vi "Init.vi"(7 "Clust Refnum":refnum<vi>, 8 "error in (no error)":errorcluster, 9 "All_info":string[][](array[string]), 10 "Path_out":string[](array[string]), 11 "Data":T1) -> (0 "error out":errorcluster, 3 "Data Out":T1)   [LabVIEW 2014]
uses:
  controls/Data1.ctl
  controls/Payjson.ctl
panel:
  in  "Save Path":string="C:\\CS-BarCode\\Save Date\\"
  in  "IO Path":path=path "C:/CS-BarCode/Setting Data/Com.ini"
  in  "Model Path":path=path "C:/CS-BarCode/Setting Data/Model.csv"
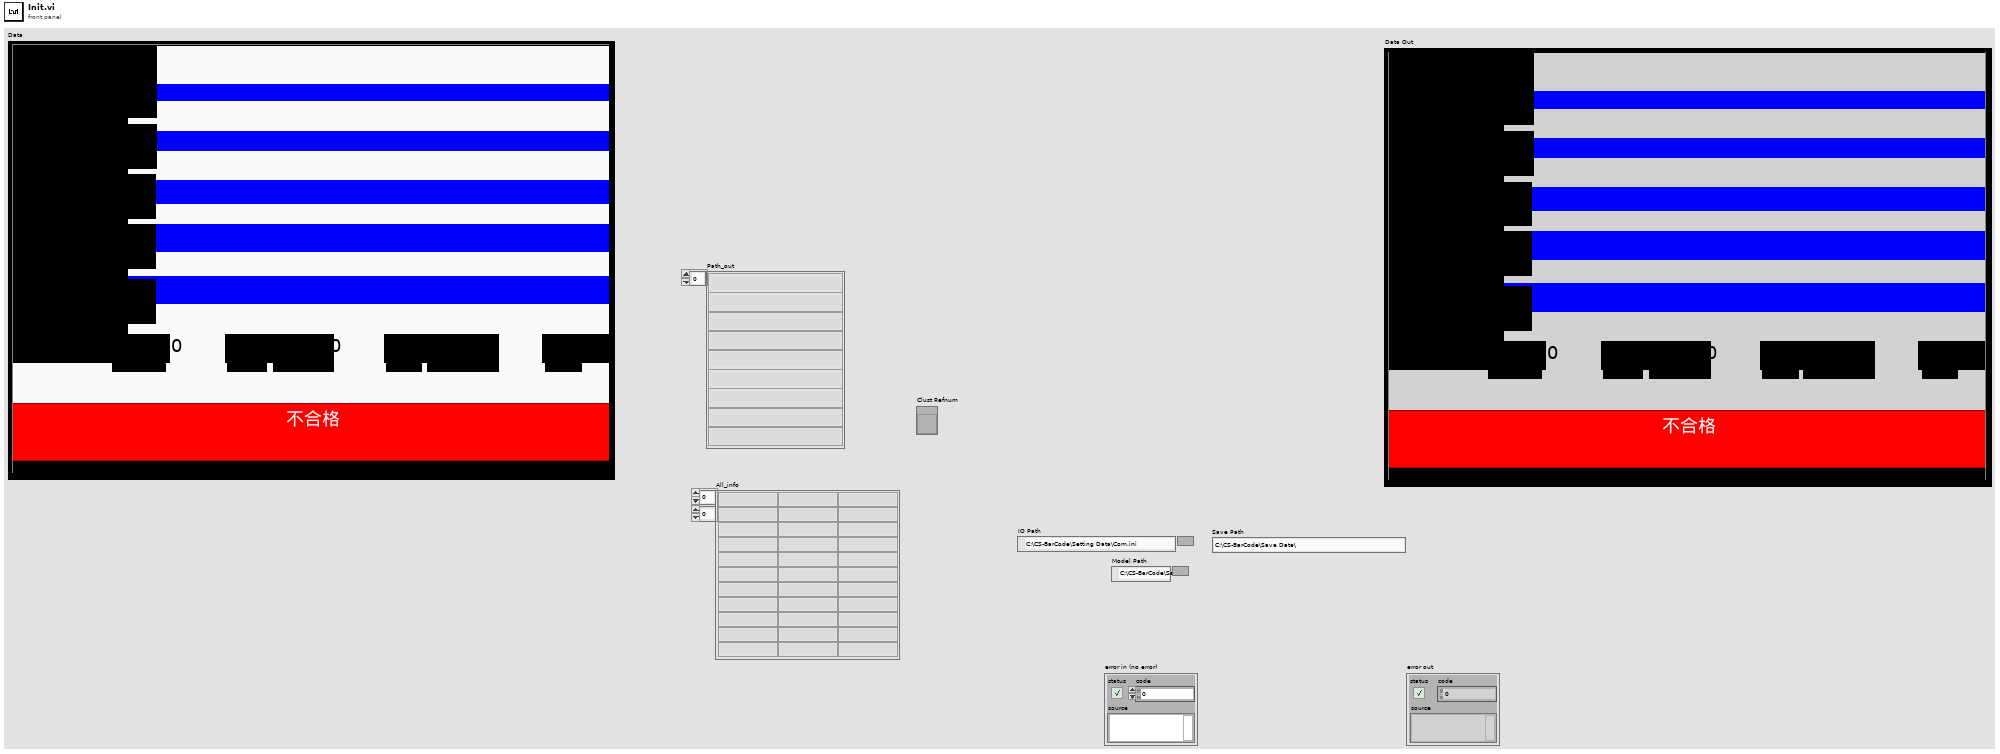
[diagram p1: front panel]
types:
  T1 = typedef "Data1.ctl" = cluster{"Date":string, "BarCode1":string, "BarCode2":string, "BarCode3":string, "Message":string, "OK Count":u16, "NG Count":u16, "Total Count":u16, "ModelData":string[][], "OK&NG":bool, "COM1":refnum<visa-resource-name>, "COM2":refnum<visa-resource-name>, "IO":i32, "Time":u32, "TCP":refnum<k5>, "TCP 2":refnum<k5>, "COM1 2":refnum<visa-resource-name>, "CheckNum":string, "BarCode1_1":string, "BarCode2_1":string, "BarCode3_1":string, "日期":string, "機種":string, "機號":string, "商品條碼1":string, "OK_1":string, "OK":string, "NG":string, "NG_1":string, "Total":string, "Total_1":string, "ClaerTime":u32, "Pjson":T2, "LotNo":string[], "CheckParsArray":string[], "BarCode4":string, "BarCode4_1":string, "商品條碼2":string, "BarCode5":string, "BarCode5_1":string, "商品條碼3":string, "ReScanNG":i32, "NGTimeCT":u32}
  T2 = typedef "Payjson.ctl" = cluster{"DEPT":string, "LINE":string, "STANO":string, "WORKNO":string, "PRODSN":string, "COMPNTID":string, "COMPNTLOT":string, "COMPNTSN":string, "USEDQTY":i16, "OPDATE":string, "OPUSER":string, "RECVDATE":string, "MMODU":string}[]
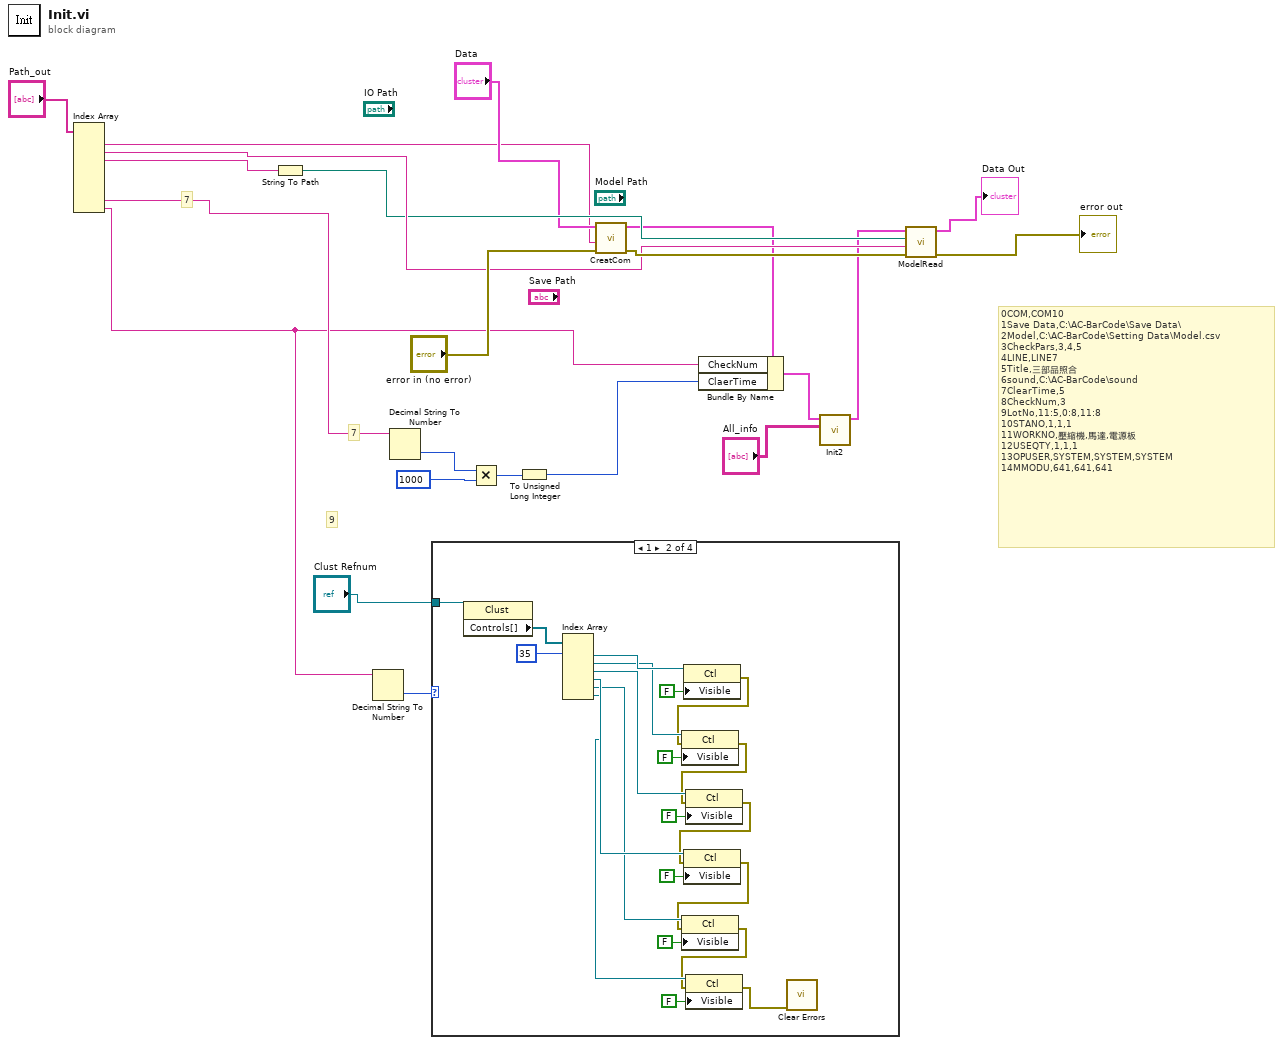
[diagram p0: block diagram]
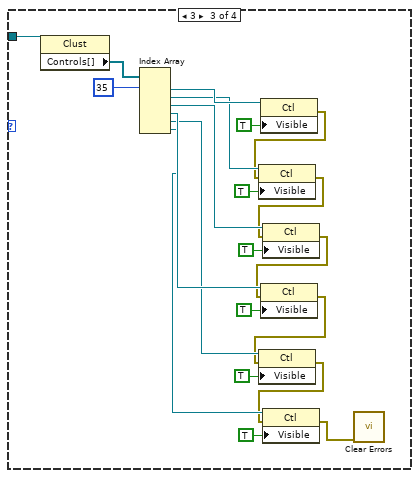
[diagram p3: hidden frame]
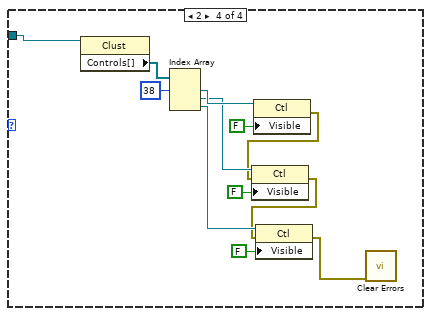
[diagram p4: hidden frame]
diagram:
  # "0COM,COM10\n1Save Data,C:\\AC-BarCode\\Save Data\\\n2Model,C:\\AC-BarCode\\Setting Data\\Model.csv\n3CheckPars,3,4,5\n4LINE,LINE7\n5Title,三部品照合\n6sound,C:\\AC-BarCode\\sound\n7ClearTime,5\n8CheckNum,3\n9LotNo,11:5,0:8,11:8\n10STANO,1,1,1\n11WORKNO,壓縮機,馬達,電源板\n12USEQTY,1,1,1\n13OPUSER,SYSTEM,SYSTEM,SYSTEM\n14MMODU,641,641,641"
  # "9"
  # "7"
  # "7"
  n1 = Index Array(array="Path_out") -> (element #1=w14:string, element #2=w18:string, element #3=w17:string, element #8=w13:string, element #9=w1:string)  [unwired: 9 in, 4 out]
  n2 = String To Path(string=w17) -> (path=w16:path)
  n3 = Decimal String To Number(string=w1) -> (number=w3:i32)  [unwired: 2 in, 1 out]
  n4 = Decimal String To Number(string=w13) -> (number=w12:i32)  [unwired: 2 in, 1 out]
  n5 = case shown="1" w3 {
    tunnel: "Clust Refnum" -> [_ w35 w56 w72]
    frame 0, Default {
    }
    frame 1 {
      n6 = property class="Clust"(reference=w35) -> ("Controls[]"=w43:refnum<vi>[])  [unwired: 1 in, 2 out]
      n7 = Index Array(array=w43, index #1=35 ("index")) -> (element #1=w41:refnum<vi>, element #2=w37:refnum<vi>, element #3=w36:refnum<vi>, element #4=w31:refnum<vi>, element #5=w30:refnum<vi>, element #6=w29:refnum<vi>)  [unwired: 5 in]
      n8 = property class="Ctl"(reference=w41, "Visible"=FALSE) -> (error out=w28:errorcluster)  [unwired: 1 in, 1 out]
      n9 = property class="Ctl"(reference=w37, error in=w28, "Visible"=FALSE) -> (error out=w27:errorcluster)  [unwired: 1 out]
      n10 = property class="Ctl"(reference=w36, error in=w27, "Visible"=FALSE) -> (error out=w26:errorcluster)  [unwired: 1 out]
      n11 = property class="Ctl"(reference=w31, error in=w26, "Visible"=FALSE) -> (error out=w25:errorcluster)  [unwired: 1 out]
      n12 = property class="Ctl"(reference=w30, error in=w25, "Visible"=FALSE) -> (error out=w24:errorcluster)  [unwired: 1 out]
      n13 = property class="Ctl"(reference=w29, error in=w24, "Visible"=FALSE) -> (error out=w23:errorcluster)  [unwired: 1 out]
      n14 = call <vilib>:"Clear Errors.vi"("error in (no error)"=w23) -> ()  [unwired: 5 in, 2 out]
    }
    frame 3 {
      n15 = property class="Clust"(reference=w56) -> ("Controls[]"=w64:refnum<vi>[])  [unwired: 1 in, 2 out]
      n16 = Index Array(array=w64, index #1=35 ("index")) -> (element #1=w62:refnum<vi>, element #2=w58:refnum<vi>, element #3=w57:refnum<vi>, element #4=w52:refnum<vi>, element #5=w51:refnum<vi>, element #6=w50:refnum<vi>)  [unwired: 5 in]
      n17 = property class="Ctl"(reference=w62, "Visible"=TRUE) -> (error out=w49:errorcluster)  [unwired: 1 in, 1 out]
      n18 = property class="Ctl"(reference=w58, error in=w49, "Visible"=TRUE) -> (error out=w48:errorcluster)  [unwired: 1 out]
      n19 = property class="Ctl"(reference=w57, error in=w48, "Visible"=TRUE) -> (error out=w47:errorcluster)  [unwired: 1 out]
      n20 = property class="Ctl"(reference=w52, error in=w47, "Visible"=TRUE) -> (error out=w46:errorcluster)  [unwired: 1 out]
      n21 = property class="Ctl"(reference=w51, error in=w46, "Visible"=TRUE) -> (error out=w45:errorcluster)  [unwired: 1 out]
      n22 = property class="Ctl"(reference=w50, error in=w45, "Visible"=TRUE) -> (error out=w44:errorcluster)  [unwired: 1 out]
      n23 = call <vilib>:"Clear Errors.vi"("error in (no error)"=w44) -> ()  [unwired: 5 in, 2 out]
    }
    frame 2 {
      n24 = property class="Clust"(reference=w72) -> ("Controls[]"=w76:refnum<vi>[])  [unwired: 1 in, 2 out]
      n25 = Index Array(array=w76, index #1=38 ("index")) -> (element #1=w74:refnum<vi>, element #2=w69:refnum<vi>, element #3=w68:refnum<vi>)  [unwired: 2 in]
      n26 = property class="Ctl"(reference=w74, "Visible"=FALSE) -> (error out=w67:errorcluster)  [unwired: 1 in, 1 out]
      n27 = property class="Ctl"(reference=w69, error in=w67, "Visible"=FALSE) -> (error out=w66:errorcluster)  [unwired: 1 out]
      n28 = property class="Ctl"(reference=w68, error in=w66, "Visible"=FALSE) -> (error out=w65:errorcluster)  [unwired: 1 out]
      n29 = call <vilib>:"Clear Errors.vi"("error in (no error)"=w65) -> ()  [unwired: 5 in, 2 out]
    }
  }
  n30 = Multiply(x=w12, y=1000) -> (x*y=w10:i32)
  n31 = To Unsigned Long Integer(number=w10) -> (unsigned 32bit integer=w9:u32)
  n32 = call "CreatCom.vi"("error in (no error)"="error in (no error)", "COM"=w14, "Data In"="Data") -> ("error out"=w22:errorcluster, "Data Out"=w6:T1)  [unwired: 7 in]
  n33 = Bundle By Name(cluster=w6, "CheckNum"=w1, "ClaerTime"=w9) -> (w7:T1)
  n34 = call "Init2.vi"("All_info"="All_info", "DataIn"=w7) -> ("DataOut"=w5:T1)  [unwired: 9 in]
  n35 = call "ModelRead.vi"("error in (no error)"=w22, "Save Path"=w18, "file path (dialog if empty)"=w16, "Data In"=w5) -> ("error out"=→"error out":errorcluster, "Data Out"=→"Data Out":T1)  [unwired: 5 in, 1 out]
